vi "rdb_json_get_element.vi"(8 "error in (no error)":errorcluster, 11 "json_dvr in":refnum<data-value>) -> (0 "error out":errorcluster, 2 "element":T1, 3 "json_dvr out":refnum<data-value>)   [LabVIEW 2017]
uses:
  rdb_json_dvr.ctl
  rdb_json_element.ctl
  rdb_json_type.ctl
panel:
  in  "key":string
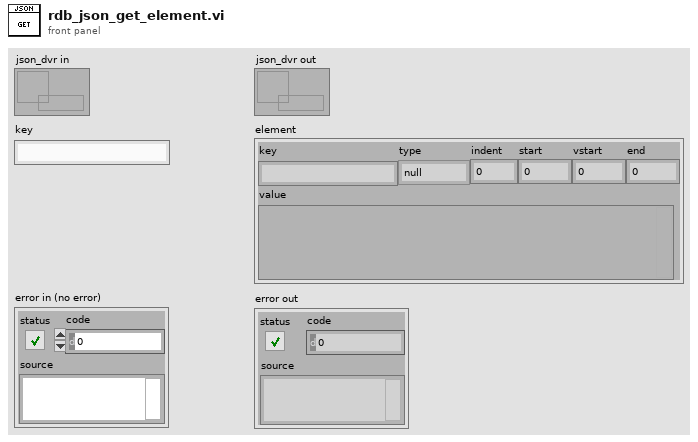
[diagram p1: front panel]
types:
  T1 = typedef "rdb_json_element.ctl" = cluster{"key":string, "type":T2, "indent":i32, "start":i32, "vstart":i32, "end":i32, "value":variant}
  T2 = typedef "rdb_json_type.ctl" = enum8{"null", "bool", "int", "uint", "float", "string", "array", "object", "invalid"}
  T3 = typedef "rdb_json_dvr.ctl" = cluster{"json":string, "elements":T1[]}
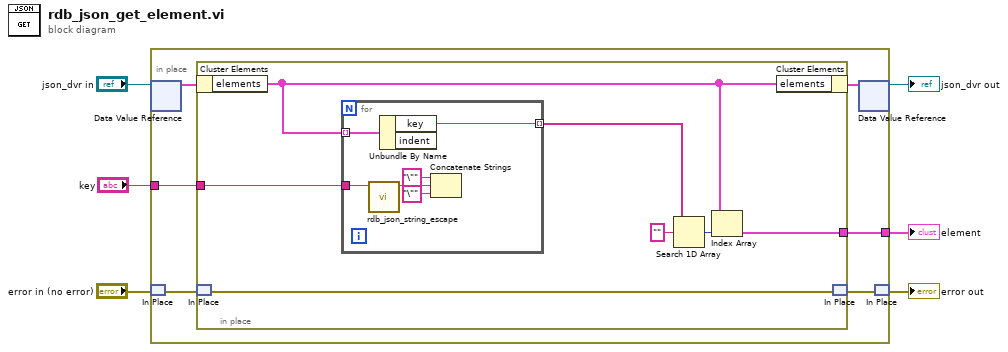
[diagram p0: block diagram]
diagram:
  n1 = in-place {
    in-place-border: [w8] -> w2
    in-place-border: "key" -> [w7]
    n2 = in-place-dvr #1("json_dvr in") -> (w10:T3)  [unwired: 1 out]
    n3 = in-place-match #2("error in (no error)") -> (w12:errorcluster)
    n4 = in-place {
      in-place-border: [w15] -> w8
      in-place-border: w7 -> [w14]
      n5 = in-place-cluster #3(w10) -> ("elements"=w17:T1[])
      n6 = in-place-match #4(w12) -> (w16:errorcluster)
      n7 = for {
        tunnel: w17 -> [w25] mode=indexing
        tunnel: [w24] -> w19 mode=indexing
        tunnel: w14 -> [w20]
        n8 = call "rdb_json_string_escape.vi"("string"=w20) -> ("escaped string"=w23:string)  [unwired: 10 in]
        n9 = Unbundle By Name(w25) -> ("key"=w24:string)  [unwired: 1 out]
        n10 = Concatenate Strings("\"" ("string"), w23, "\"" ("string")) -> ()  [unwired: 1 out]
      }
      n11 = Search 1D Array(1D array=w19, element="") -> (index of element=w18:i32)  [unwired: 1 in]
      n12 = Index Array(array=w17, index=w18) -> (element=w15:T1)
      n13 = in-place-cluster #3("elements"=w17) -> (w9:T3)
      n14 = in-place-match #4(w16) -> (w11:errorcluster)
    }
    n15 = in-place-dvr #1(w9) -> (→"json_dvr out":refnum<data-value>)  [unwired: 1 out]
    n16 = in-place-match #2(w11) -> (→"error out":errorcluster)
  }
  "element" <- w2
